vi "Read State.vi"(8 "error in":errorcluster, 11 "DAQmxSwitch in":refnum<class "DAQmxSwitch.lvclass">) -> (0 "error out":errorcluster, 2 "State":bool, 3 "DAQmxSwitch out":refnum<class "DAQmxSwitch.lvclass">)   [LabVIEW 2014, in "DAQmxSwitch.lvclass"]
uses:
  DAQmxSwitch.lvclass
  <resource>/objmgr/daqmx.rc
  <vilib>/DAQmx/read.llb/DAQmx Read (Digital 1D Bool NChan 1Samp 1Line).vi
  <vilib>/DAQmx/read.llb/DAQmx Read (Digital Bool 1Line 1Point).vi
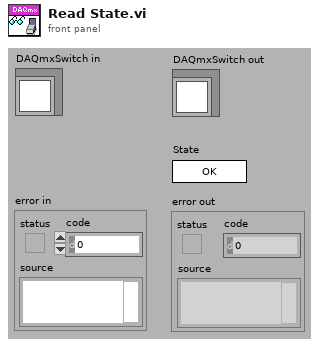
[diagram p1: front panel]
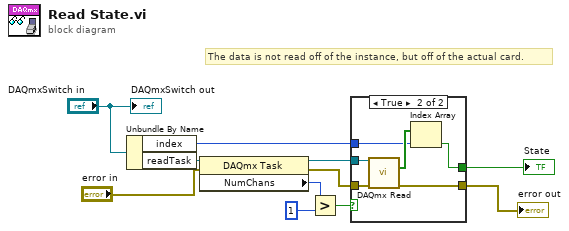
[diagram p0: block diagram]
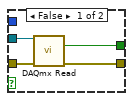
[diagram p2: hidden frame]
diagram:
  # "The data is not read off of the instance, but off of the actual card."
  n1 = Unbundle By Name("DAQmxSwitch in") -> ("index"=w6:i32, "readTask"=w11:refnum<k21>)
  n2 = property class="DAQmx Task"(reference=w11, error in="error in") -> (reference out=w9:refnum<k21>, error out=w5:errorcluster, "NumChans"=w10:u32)
  n3 = Greater?(x=w10, y=u32 1) -> (0:w7:bool)
  n4 = case shown="True" w7 {
    tunnel: w9 -> [w15 w21]
    tunnel: w5 -> [w14 w20]
    tunnel: w6 -> [_ w16]
    tunnel: [w12 w18] -> w1
    tunnel: [w13 w17] -> w3
    frame False {
      n5 = call-poly <vilib>:"DAQmx Read.vi"("task/channels in"=w15, "error in"=w14) -> ("data"=w13:bool, "error out"=w12:errorcluster)  [unwired: 11 in, 1 out]
    }
    frame True {
      n6 = call-poly <vilib>:"DAQmx Read.vi"("task/channels in"=w21, "error in"=w20) -> ("data"=w19:bool[], "error out"=w18:errorcluster)  [unwired: 11 in, 1 out]
      n7 = Index Array(array=w19, index=w16) -> (element=w17:bool)
    }
  }
  "error out" <- w1
  "State" <- w3
  "DAQmxSwitch out" <- "DAQmxSwitch in"
